vi "Get Target_Dest_Path.vi"(8 "error in (no error)":errorcluster, 11 "AB_Build in":refnum<class "AB_Build.lvclass">) -> (0 "error out":errorcluster, 2 "Target Dest Path":path, 3 "AB_Build out":refnum<class "AB_Build.lvclass">)   [LabVIEW 2020, in "AB_Build.lvclass"]
uses:
  <vilib>/AppBuilder/AB_Classes/Build/AB_Build.lvclass
  <vilib>/AppBuilder/AB_Classes/Build/AB_Build.lvclass/AB_Build.ctl
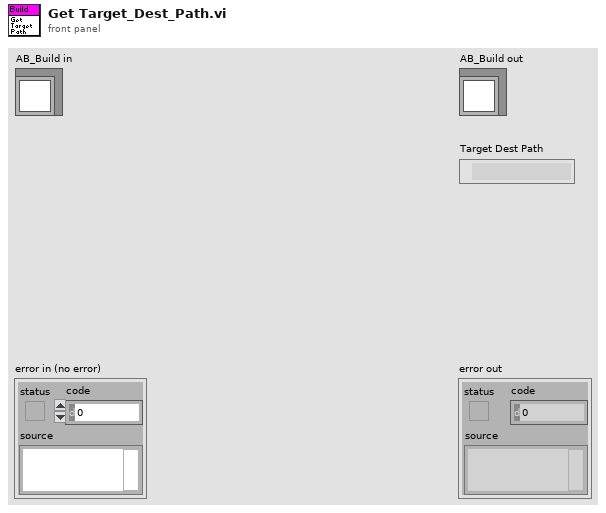
[diagram p1: front panel]
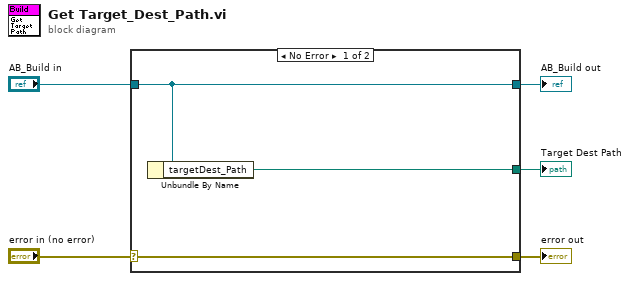
[diagram p0: block diagram]
diagram:
  n1 = case shown="No Error" "error in (no error)" {
    selector: "error in (no error)" -> [w8 w9]
    tunnel: [w8 w9] -> w4
    tunnel: [w7 w10] -> w2
    tunnel: "AB_Build in" -> [w7 w10]
    tunnel: [w6 _] -> w1
    frame No Error {
      n2 = Unbundle By Name(w7) -> ("targetDest_Path"=w6:path)
    }
    frame Error {
    }
  }
  "error out" <- w4
  "AB_Build out" <- w2
  "Target Dest Path" <- w1
